vi "2-7.vi"() -> ()   [LabVIEW 2022 SP3]
panel:
  out "第3列的元素":dbl[](array[numeric])
  out "第0行的元素":dbl[](array[numeric])
  out "第2行第1列元素":dbl
  out "数组大小":dbl[](array[numeric])
  out "数组":dbl[][](array[numeric])
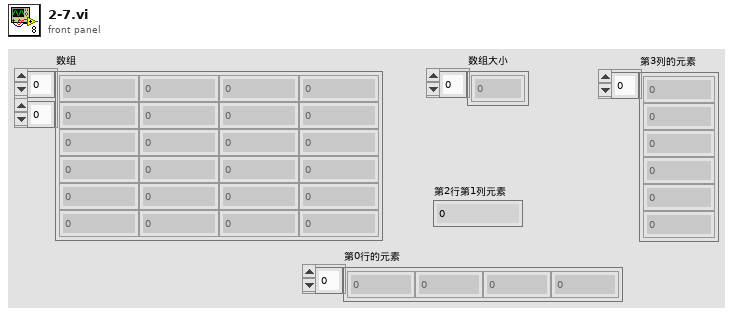
[diagram p1: front panel]
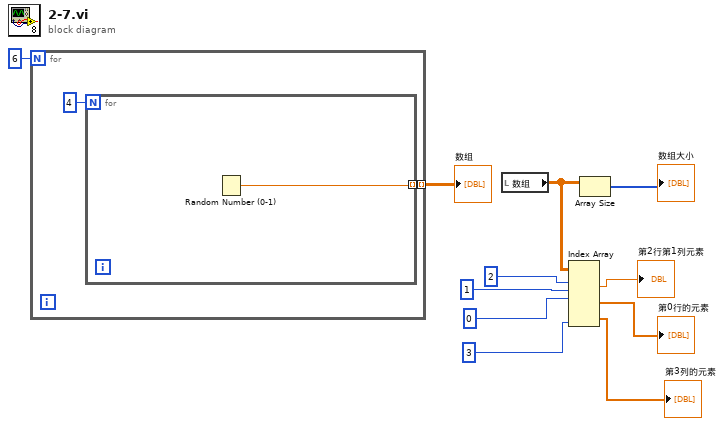
[diagram p0: block diagram]
diagram:
  n1 = for {
    N: 6 -> [_]
    tunnel: [w13] -> w10 mode=indexing
    n2 = for {
      N: 4 -> [_]
      tunnel: [w14] -> w13 mode=indexing
      n3 = Random Number (0-1)() -> (number: 0 to 1=w14:dbl)
    }
  }
  "数组" <- w10
  n4 = local read "数组"() -> (w4:dbl[][])
  n5 = Index Array(array=w4, index (row) #1=2, index (col) #1=1, index (row) #2=0, index (col) #3=3) -> (element #1=→"第2行第1列元素":dbl, element #2=→"第0行的元素":dbl[], element #3=→"第3列的元素":dbl[])  [unwired: 2 in]
  n6 = Array Size(array=w4) -> (size(s)=→"数组大小":i32[])
